vi "has_current.vi"(8 "error in (no error)":errorcluster, 11 "Application in":refnum<vi>) -> (0 "error out":errorcluster, 2 "Boolean":bool, 3 "Application out":refnum<vi>)   [LabVIEW 2014]
uses:
  <userlib>/Nanonis Prog Interface V5/Nanonis Prog Interface.lvlib
panel:
  in  "current threshold":sgl=2e-11 format="%#_6p"
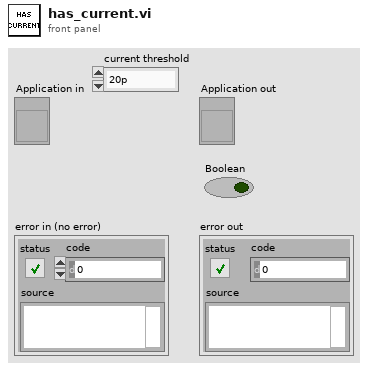
[diagram p1: front panel]
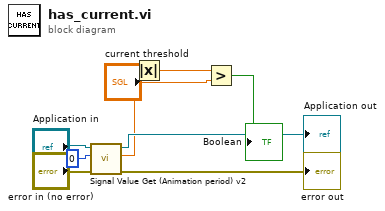
[diagram p0: block diagram]
diagram:
  n1 = call <userlib>:"Signal Value Get (Animation period) v2.vi"("error in (no error)"="error in (no error)", "Signal index (0-79)"=i8 0, "Application ref in"="Application in") -> ("error out"=→"error out":errorcluster, "Signal value"=w4:sgl, "Application ref out"=→"Application out":refnum<vi>)  [unwired: 5 in]
  n2 = Absolute Value(x=w4) -> (abs(x)=w6:sgl)
  n3 = Greater?(x=w6, y="current threshold") -> (0:→"Boolean":bool)
